vi "ProcessData.vi"(8 "error in (no error)":errorcluster, 9 "State":T1, 10 "Analog Data":T3, 11 "PassiveFixation in":refnum<class "PassiveFixation.lvclass">) -> (0 "error out":errorcluster, 1 "Fixated":bool, 2 "Trigger":T2=enum."Broke Fixation", 3 "PassiveFixation out":refnum<class "PassiveFixation.lvclass">)   [LabVIEW 2010, in "PassiveFixation.lvclass"]
uses:
  PassiveFixation.lvclass
  Core SubVIs/Controls/TYPE - Analog Data.ctl
  Trial Based Experiment.lvsc/Trigger.ctl
  Trial Based Experiment.lvsc/State.ctl
  <vilib>/measure/madcrms.llb/Basic Averaged DC-RMS for 1 Chan.vi
  Core SubVIs/Core SubVIs.lvlib
  <vilib>/measure/NI_MAPro.lvlib
  Trial Based Experiment.lvsc
panel:
  in  "Adjustment Rate":dbl=0.02
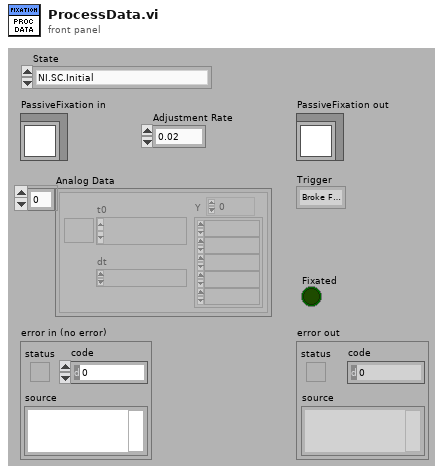
[diagram p1: front panel]
types:
  T1 = typedef "Trial Based Experiment.lvsc/State.ctl" = enum16{"NI.SC.Initial", "NI.SC.History", "NI.SC.ShallowHistory", "NI.SC.Terminal", "Cleanup", "State", "State\\Region\\Pause", "State\\Region\\Response Period", "State\\Region\\Delay Period", "State\\Region\\Hold Fixation", "State\\Region\\Acquire Fixation", "State\\Region\\Abort Trial", "State\\Region\\End Trial", "State\\Region\\Intertrial", "State\\Region\\Start Trial"}
  T2 = typedef "Trial Based Experiment.lvsc/Trigger.ctl" = enum16{"NULL", "Fixated", "Broke Fixation", "Stop", "Correct Response", "Incorrect Response", "Timeout"}
  T3 = typedef "Core SubVIs.lvlib/TYPE - Analog Data.ctl" = waveform(dbl)[]
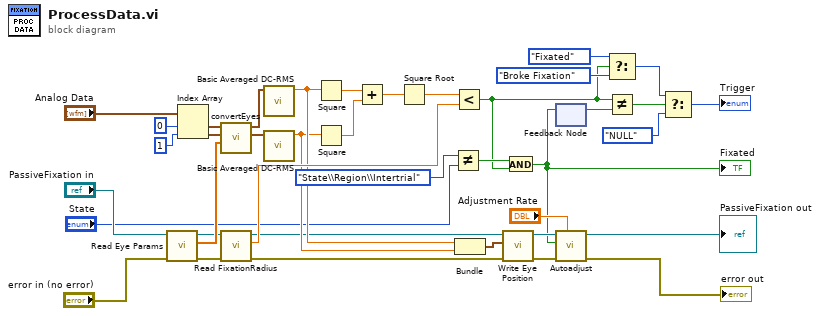
[diagram p0: block diagram]
diagram:
  n1 = call-dynamic "Read Eye Params.vi"("error in (no error)"="error in (no error)", "TrialBasedExperiment in"="PassiveFixation in") -> ("error out"=w16:errorcluster, "Eye Params"=w34:dbl[], "TrialBasedExperiment out"=w17:refnum<class "PassiveFixation.lvclass">)  [unwired: 7 in]
  n2 = Index Array(array="Analog Data", index #1=0 ("index"), index #2=1 ("index")) -> (element #1=w32:waveform(dbl), element #2=w31:waveform(dbl))
  n3 = call "convertEyes.vi"("Params"=w34, "Vertical"=w31, "Horizontal"=w32) -> ("Vertical Calibrated"=w37:waveform(dbl), "Horizontal Calibrated"=w36:waveform(dbl))  [unwired: 7 in]
  n4 = call-dynamic "Read FixationRadius.vi"("error in (no error)"=w16, "MatlabExperiment in"=w17) -> ("error out"=w8:errorcluster, "FixationRadius"=w18:dbl, "MatlabExperiment out"=w12:refnum<class "PassiveFixation.lvclass">)  [unwired: 7 in]
  n5 = call-poly <vilib>:"Basic Averaged DC-RMS.vi"("signal in"=w36) -> ("DC value"=w15:dbl)  [unwired: 7 in, 3 out]
  n6 = call-poly <vilib>:"Basic Averaged DC-RMS.vi"("signal in"=w37) -> ("DC value"=w14:dbl)  [unwired: 7 in, 3 out]
  n7 = Square(x=w15) -> (x^2=w26:dbl)
  n8 = Square(x=w14) -> (x^2=w25:dbl)
  n9 = Add(x=w26, y=w25) -> (x+y=w24:dbl)
  n10 = Square Root(x=w24) -> (sqrt(x)=w23:dbl)
  n11 = Not Equal?(x=State."State\\Region\\Intertrial", y="State") -> (x != y?=w3:bool)
  n12 = Less?(x=w23, y=w18) -> (x < y?=w2:bool)
  n13 = Bundle("DC value"=w15, "DC value"=w14) -> (w13:cluster{"DC value":dbl, "DC value":dbl})  [unwired: 1 in]
  n14 = call-dynamic "Write Eye Position.vi"("error in (no error)"=w8, "Eye Position"=w13, "TrialBasedExperiment in"=w12) -> ("error out"=w7:errorcluster, "TrialBasedExperiment out"=w11:refnum<class "PassiveFixation.lvclass">)  [unwired: 7 in]
  n15 = And(x=w3, y=w2) -> (x .and. y?=w1:bool)
  "Fixated" <- w1
  n16 = feedback #1() -> (w27:bool)  [unwired: 1 in]
  n17 = feedback-in #1(w1) -> ()
  n18 = call-dynamic "Autoadjust.vi"("Adjustment Rate"="Adjustment Rate", "error in (no error)"=w7, "Fixated"=w1, "TrialBasedExperiment in"=w11) -> ("error out"=→"error out":errorcluster, "TrialBasedExperiment out"=→"PassiveFixation out":refnum<class "PassiveFixation.lvclass">)  [unwired: 6 in]
  n19 = Select(t=Trigger."Fixated" ("Trigger"), s=w2, f=Trigger."Broke Fixation" ("Trigger")) -> (s? t:f=w28:T2)
  n20 = Not Equal?(x=w2, y=w27) -> (x != y?=w20:bool)
  n21 = Select(t=w28, s=w20, f=Trigger."NULL" ("Trigger")) -> (s? t:f=→"Trigger":T2)
